vi "4bar setpoint and immediate.vi"(6 "Operator X Button":bool, 8 "Operator Y Button":bool, 9 "Operator B Button":bool, 10 "Operator A Button":bool, 11 "Operator Right Joystick Y in":dbl) -> (3 "Output":T2 {"Control Mode" items=["PercentOutput"=0, "Position"=1, "Velocity"=2, "Current"=3, "Follower"=5, "MotionProfile"=6, "MotionMagic"=7, "MotionProfileArc"=10, "Disabled"=15]})   [LabVIEW 2018]
uses:
  <vilib>/Rock Robotics/WPI/ThirdParty/Phoenix-LabVIEW/Motor Controller/Controls/CTRE_Phoenix_MotorControl_ControlMode.ctl
  4barCommands.ctl
  Infrastructure/Constants.vi
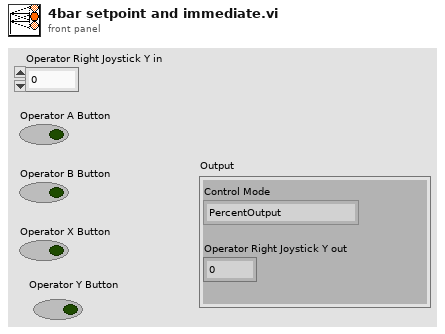
[diagram p1: front panel]
types:
  T1 = typedef "CTRE_Phoenix_MotorControl_ControlMode.ctl" = u16
  T2 = cluster{"Control Mode":T1, "Operator Right Joystick Y out":dbl}
  T3 = typedef "4barCommands.ctl" = enum16{"Immediate", "Hold", "Setpoint"}
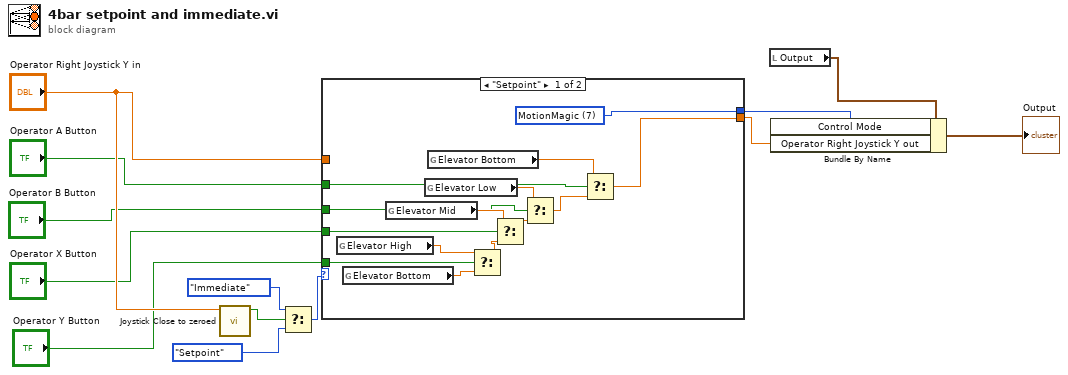
[diagram p0: block diagram]
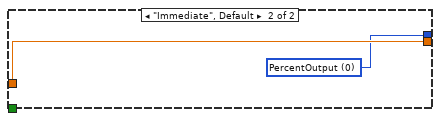
[diagram p2: hidden frame]
diagram:
  n1 = call "Joystick Close to zeroed.vi"("Joystick"="Operator Right Joystick Y in") -> ("=0?"=w12:bool)  [unwired: 10 in]
  n2 = Select(t=4barCommands."Immediate", s=w12, f=4barCommands."Setpoint") -> (s? t:f=w10:T3)
  n3 = case shown="\"Setpoint\"" w10 {
    tunnel: "Operator X Button" -> [w22 _]
    tunnel: "Operator B Button" -> [w21 _]
    tunnel: "Operator A Button" -> [w20 _]
    tunnel: "Operator Right Joystick Y in" -> [_ w29]
    tunnel: [w19 w28] -> w4
    tunnel: [w18 w29] -> w3
    tunnel: "Operator Y Button" -> [w16 _]
    frame "Setpoint" {
      w19 = T1 7 items=["PercentOutput"=0, "Position"=1, "Velocity"=2, "Current"=3, "Follower"=5, "MotionProfile"=6, "MotionMagic"=7, "MotionProfileArc"=10, "Disabled"=15] ("Control Mode")
      n4 = global read "Constants.vi" "Elevator High"() -> (w17:dbl)
      n5 = global read "Constants.vi" "Elevator Bottom"() -> (w15:dbl)
      n6 = global read "Constants.vi" "Elevator Mid"() -> (w25:dbl)
      n7 = global read "Constants.vi" "Elevator Low"() -> (w24:dbl)
      n8 = global read "Constants.vi" "Elevator Bottom"() -> (w23:dbl)
      n9 = Select(t=w17, s=w16, f=w15) -> (s? t:f=w14:dbl)
      n10 = Select(t=w25, s=w22, f=w14) -> (s? t:f=w26:dbl)
      n11 = Select(t=w24, s=w21, f=w26) -> (s? t:f=w27:dbl)
      n12 = Select(t=w23, s=w20, f=w27) -> (s? t:f=w18:dbl)
    }
    frame "Immediate", Default {
      w28 = T1 0 items=["PercentOutput"=0, "Position"=1, "Velocity"=2, "Current"=3, "Follower"=5, "MotionProfile"=6, "MotionMagic"=7, "MotionProfileArc"=10, "Disabled"=15] ("Control Mode")
    }
  }
  n13 = local read "Output"() -> (w1:T2)
  n14 = Bundle By Name(cluster=w1, "Control Mode"=w4, "Operator Right Joystick Y out"=w3) -> (→"Output":T2)
